vi "CylinderIRQ_EPTx.vi"(8 "IRQControls":T1(array[cluster])=[{"Enable"=FALSE, "IRQ CAD"=0.0, "IRQ Window Start"=0.0, "IRQ Window End"=0.0}, {"Enable"=FALSE, "IRQ CAD"=0.0, "IRQ Window Start"=0.0, "IRQ Window End"=0.0}, {"Enable"=FALSE, "IRQ CAD"=0.0, "IRQ Window Start"=0.0, "IRQ Window End"=0.0}, {"Enable"=FALSE, "IRQ CAD"=0.0, "IRQ Window Start"=0.0, "IRQ Window End"=0.0}, {"Enable"=FALSE, "IRQ CAD"=0.0, "IRQ Window Start"=0.0, "IRQ Window End"=0.0}, {"Enable"=FALSE, "IRQ CAD"=0.0, "IRQ Window Start"=0.0, "IRQ Window End"=0.0}, {"Enable"=FALSE, "IRQ CAD"=0.0, "IRQ Window Start"=0.0, "IRQ Window End"=0.0}, {"Enable"=FALSE, "IRQ CAD"=0.0, "IRQ Window Start"=0.0, "IRQ Window End"=0.0}], 11 "EPTxSupervisor":T2) -> ()   [LabVIEW 2015, in "ECS-FPGA.lvlib"]
uses:
  ECS-FPGA.lvlib
  <vilib>/Powertrain Controls/Device Drivers/Engine Position Tracking/EPTx/RevA/FPGA/Controls/EPTxSupervisor.ctl
  <vilib>/Powertrain Controls/Device Drivers/Engine Position Tracking/EPTx/RevA/FPGA/Controls/EPTxAOSControl.ctl
  <vilib>/Powertrain Controls/Device Drivers/Engine Position Tracking/EPTx/RevA/FPGA/Controls/EPTxAAPControl.ctl
  <vilib>/Powertrain Controls/Device Drivers/Engine Position Tracking/EPTx/RevA/FPGA/EPTx - RevA - FPGA.lvlib
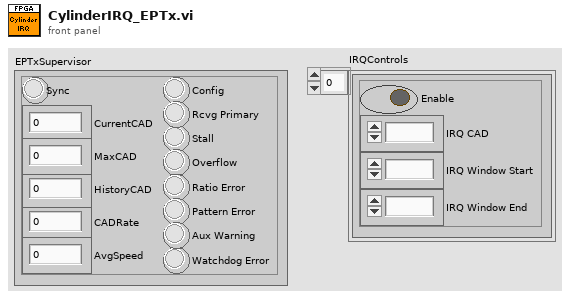
[diagram p1: front panel]
types:
  T1 = cluster{"Enable":bool, "IRQ CAD":fxp<+,18,11>, "IRQ Window Start":fxp<+,18,11>, "IRQ Window End":fxp<+,18,11>}[]
  T2 = typedef "EPTx - RevA - FPGA.lvlib/EPTxSupervisor.ctl" = cluster{"Sync":bool, "CurrentCAD":fxp<+,18,11>, "MaxCAD":fxp<+,11,11>, "HistoryCAD":fxp<+,11,11>, "CADRate":fxp<+,22,8>, "AvgSpeed":fxp<+,17,15>, "Config":bool, "Rcvg Primary":bool, "Stall":bool, "Overflow":bool, "Ratio Error":bool, "Pattern Error":bool, "Aux Warning":bool, "Watchdog Error":bool}
  T3 = typedef "EPTx - RevA - FPGA.lvlib/EPTxAAPControl.ctl" = cluster{"Enable":bool, "RisingCAD":fxp<+,18,11>, "FallingCAD":fxp<+,18,11>}
  T4 = typedef "EPTx - RevA - FPGA.lvlib/EPTxAOSControl.ctl" = cluster{"Enable":bool, "OneShotCAD":fxp<+,18,11>}
  T5 = cluster{"Enable":bool, "IRQ CAD":fxp<+,18,11>, "IRQ Window Start":fxp<+,18,11>, "IRQ Window End":fxp<+,18,11>}
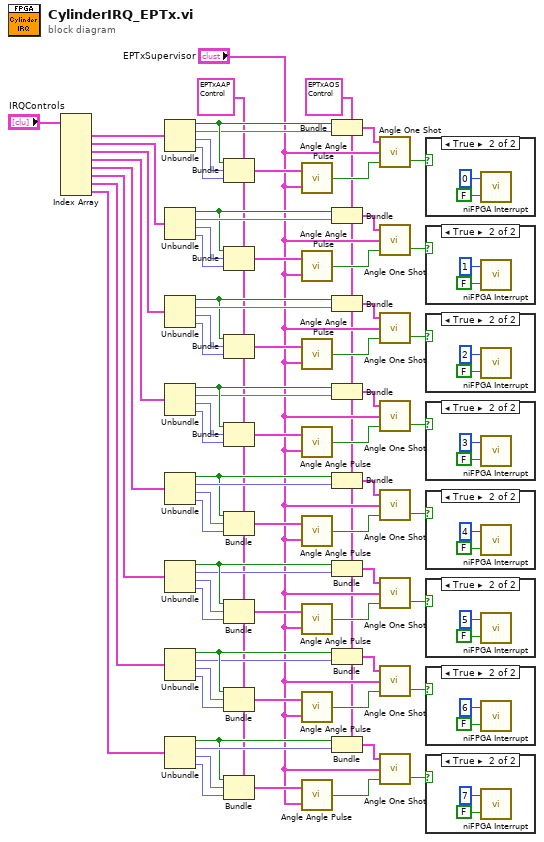
[diagram p0: block diagram]
diagram:
  w3 = T3 {"Enable"=FALSE, "RisingCAD"=0.0, "FallingCAD"=0.0} ("AAPControl")
  w1 = T4 {"Enable"=FALSE, "OneShotCAD"=0.0} ("AOSControl")
  n1 = Index Array(array="IRQControls") -> (element #1=w67:T5, element #2=w58:T5, element #3=w41:T5, element #4=w40:T5, element #5=w7:T5, element #6=w6:T5, element #7=w5:T5, element #8=w4:T5)  [unwired: 8 in]
  n2 = Unbundle(w67) -> ("Enable"=w72:bool, "IRQ CAD"=w71:fxp<+,18,11>, "IRQ Window Start"=w70:fxp<+,18,11>, "IRQ Window End"=w69:fxp<+,18,11>)
  n3 = Unbundle(w58) -> ("Enable"=w63:bool, "IRQ CAD"=w64:fxp<+,18,11>, "IRQ Window Start"=w65:fxp<+,18,11>, "IRQ Window End"=w66:fxp<+,18,11>)
  n4 = Unbundle(w41) -> ("Enable"=w46:bool, "IRQ CAD"=w47:fxp<+,18,11>, "IRQ Window Start"=w48:fxp<+,18,11>, "IRQ Window End"=w49:fxp<+,18,11>)
  n5 = Unbundle(w40) -> ("Enable"=w53:bool, "IRQ CAD"=w52:fxp<+,18,11>, "IRQ Window Start"=w51:fxp<+,18,11>, "IRQ Window End"=w50:fxp<+,18,11>)
  n6 = Unbundle(w7) -> ("Enable"=w12:bool, "IRQ CAD"=w13:fxp<+,18,11>, "IRQ Window Start"=w14:fxp<+,18,11>, "IRQ Window End"=w15:fxp<+,18,11>)
  n7 = Unbundle(w6) -> ("Enable"=w19:bool, "IRQ CAD"=w18:fxp<+,18,11>, "IRQ Window Start"=w17:fxp<+,18,11>, "IRQ Window End"=w16:fxp<+,18,11>)
  n8 = Unbundle(w5) -> ("Enable"=w35:bool, "IRQ CAD"=w34:fxp<+,18,11>, "IRQ Window Start"=w33:fxp<+,18,11>, "IRQ Window End"=w32:fxp<+,18,11>)
  n9 = Unbundle(w4) -> ("Enable"=w28:bool, "IRQ CAD"=w29:fxp<+,18,11>, "IRQ Window Start"=w30:fxp<+,18,11>, "IRQ Window End"=w31:fxp<+,18,11>)
  n10 = Bundle(cluster=w3, "Enable"=w72, "RisingCAD"=w70, "FallingCAD"=w69) -> (w76:T3)
  n11 = Bundle(cluster=w3, "Enable"=w63, "RisingCAD"=w65, "FallingCAD"=w66) -> (w59:T3)
  n12 = Bundle(cluster=w3, "Enable"=w46, "RisingCAD"=w48, "FallingCAD"=w49) -> (w42:T3)
  n13 = Bundle(cluster=w3, "Enable"=w53, "RisingCAD"=w51, "FallingCAD"=w50) -> (w57:T3)
  n14 = Bundle(cluster=w3, "Enable"=w12, "RisingCAD"=w14, "FallingCAD"=w15) -> (w8:T3)
  n15 = Bundle(cluster=w3, "Enable"=w19, "RisingCAD"=w17, "FallingCAD"=w16) -> (w23:T3)
  n16 = Bundle(cluster=w3, "Enable"=w35, "RisingCAD"=w33, "FallingCAD"=w32) -> (w39:T3)
  n17 = Bundle(cluster=w3, "Enable"=w28, "RisingCAD"=w30, "FallingCAD"=w31) -> (w24:T3)
  n18 = call <vilib>:"Angle Angle Pulse.vi"("EPTxSupervisor"="EPTxSupervisor", "AAPControl"=w76) -> ("AAP"=w74:bool)
  n19 = call <vilib>:"Angle Angle Pulse.vi"("EPTxSupervisor"="EPTxSupervisor", "AAPControl"=w59) -> ("AAP"=w61:bool)
  n20 = call <vilib>:"Angle Angle Pulse.vi"("EPTxSupervisor"="EPTxSupervisor", "AAPControl"=w42) -> ("AAP"=w44:bool)
  n21 = call <vilib>:"Angle Angle Pulse.vi"("EPTxSupervisor"="EPTxSupervisor", "AAPControl"=w57) -> ("AAP"=w55:bool)
  n22 = call <vilib>:"Angle Angle Pulse.vi"("EPTxSupervisor"="EPTxSupervisor", "AAPControl"=w8) -> ("AAP"=w10:bool)
  n23 = call <vilib>:"Angle Angle Pulse.vi"("EPTxSupervisor"="EPTxSupervisor", "AAPControl"=w23) -> ("AAP"=w21:bool)
  n24 = call <vilib>:"Angle Angle Pulse.vi"("EPTxSupervisor"="EPTxSupervisor", "AAPControl"=w39) -> ("AAP"=w37:bool)
  n25 = call <vilib>:"Angle Angle Pulse.vi"("EPTxSupervisor"="EPTxSupervisor", "AAPControl"=w24) -> ("AAP"=w26:bool)
  n26 = Bundle(cluster=w1, "Enable"=w72, "OneShotCAD"=w71) -> (w75:T4)
  n27 = Bundle(cluster=w1, "Enable"=w63, "OneShotCAD"=w64) -> (w60:T4)
  n28 = Bundle(cluster=w1, "Enable"=w46, "OneShotCAD"=w47) -> (w43:T4)
  n29 = Bundle(cluster=w1, "Enable"=w53, "OneShotCAD"=w52) -> (w56:T4)
  n30 = Bundle(cluster=w1, "Enable"=w12, "OneShotCAD"=w13) -> (w9:T4)
  n31 = Bundle(cluster=w1, "Enable"=w19, "OneShotCAD"=w18) -> (w22:T4)
  n32 = Bundle(cluster=w1, "Enable"=w35, "OneShotCAD"=w34) -> (w38:T4)
  n33 = Bundle(cluster=w1, "Enable"=w28, "OneShotCAD"=w29) -> (w25:T4)
  n34 = call <vilib>:"Angle One Shot.vi"("OpWindow"=w74, "EPTxSupervisor"="EPTxSupervisor", "AOSControl"=w75) -> ("AOS"=w73:bool)  [unwired: 1 in]
  n35 = call <vilib>:"Angle One Shot.vi"("OpWindow"=w61, "EPTxSupervisor"="EPTxSupervisor", "AOSControl"=w60) -> ("AOS"=w62:bool)  [unwired: 1 in]
  n36 = call <vilib>:"Angle One Shot.vi"("OpWindow"=w44, "EPTxSupervisor"="EPTxSupervisor", "AOSControl"=w43) -> ("AOS"=w45:bool)  [unwired: 1 in]
  n37 = call <vilib>:"Angle One Shot.vi"("OpWindow"=w55, "EPTxSupervisor"="EPTxSupervisor", "AOSControl"=w56) -> ("AOS"=w54:bool)  [unwired: 1 in]
  n38 = call <vilib>:"Angle One Shot.vi"("OpWindow"=w10, "EPTxSupervisor"="EPTxSupervisor", "AOSControl"=w9) -> ("AOS"=w11:bool)  [unwired: 1 in]
  n39 = call <vilib>:"Angle One Shot.vi"("OpWindow"=w21, "EPTxSupervisor"="EPTxSupervisor", "AOSControl"=w22) -> ("AOS"=w20:bool)  [unwired: 1 in]
  n40 = call <vilib>:"Angle One Shot.vi"("OpWindow"=w37, "EPTxSupervisor"="EPTxSupervisor", "AOSControl"=w38) -> ("AOS"=w36:bool)  [unwired: 1 in]
  n41 = call <vilib>:"Angle One Shot.vi"("OpWindow"=w26, "EPTxSupervisor"="EPTxSupervisor", "AOSControl"=w25) -> ("AOS"=w27:bool)  [unwired: 1 in]
  n42 = case shown="True" w73 {
    frame False {
    }
    frame True {
      n43 = call <vilib>:"niFPGA Interrupt.vi"("Wait Until Cleared (F)"=FALSE, "IRQ Number (0)"=u8 0) -> ()  [unwired: 1 in]
    }
  }
  n44 = case shown="True" w62 {
    frame False {
    }
    frame True {
      n45 = call <vilib>:"niFPGA Interrupt.vi"("Wait Until Cleared (F)"=FALSE, "IRQ Number (0)"=u8 1) -> ()  [unwired: 1 in]
    }
  }
  n46 = case shown="True" w45 {
    frame False {
    }
    frame True {
      n47 = call <vilib>:"niFPGA Interrupt.vi"("Wait Until Cleared (F)"=FALSE, "IRQ Number (0)"=u8 2) -> ()  [unwired: 1 in]
    }
  }
  n48 = case shown="True" w54 {
    frame False {
    }
    frame True {
      n49 = call <vilib>:"niFPGA Interrupt.vi"("Wait Until Cleared (F)"=FALSE, "IRQ Number (0)"=u8 3) -> ()  [unwired: 1 in]
    }
  }
  n50 = case shown="True" w11 {
    frame False {
    }
    frame True {
      n51 = call <vilib>:"niFPGA Interrupt.vi"("Wait Until Cleared (F)"=FALSE, "IRQ Number (0)"=u8 4) -> ()  [unwired: 1 in]
    }
  }
  n52 = case shown="True" w20 {
    frame False {
    }
    frame True {
      n53 = call <vilib>:"niFPGA Interrupt.vi"("Wait Until Cleared (F)"=FALSE, "IRQ Number (0)"=u8 5) -> ()  [unwired: 1 in]
    }
  }
  n54 = case shown="True" w36 {
    frame False {
    }
    frame True {
      n55 = call <vilib>:"niFPGA Interrupt.vi"("Wait Until Cleared (F)"=FALSE, "IRQ Number (0)"=u8 6) -> ()  [unwired: 1 in]
    }
  }
  n56 = case shown="True" w27 {
    frame False {
    }
    frame True {
      n57 = call <vilib>:"niFPGA Interrupt.vi"("Wait Until Cleared (F)"=FALSE, "IRQ Number (0)"=u8 7) -> ()  [unwired: 1 in]
    }
  }
